vi "Generate Target Compatibility Report.vi"(8 "Error In":errorcluster, 11 "Install LV Data":T2={"SSH Session"=refnum, "Status Log"="", "Detailed Log"="", "Credentials"={"Hostname or IP"="192.168.7.2", "Username"="root", "Password"=""}, "Target Info"={"OS Version"="", "CPU"="", "Systemd Version"="", "Internet Access"=FALSE, "Device Type"="", "LV Installed Ver"="", "LV Available Ver"="", "LV Upgrade Available"=FALSE, "Hostname"="", "NIC Info"=[]}, "Reboot Required?"=FALSE}) -> (0 "Error Out":errorcluster, 1 "Can Continue?":bool, 2 "Warnings":T1[](array[typedef]), 3 "Install LV Data":T2={"SSH Session"=refnum, "Status Log"="", "Detailed Log"="", "Credentials"={"Hostname or IP"="192.168.7.2", "Username"="root", "Password"=""}, "Target Info"={"OS Version"="", "CPU"="", "Systemd Version"="", "Internet Access"=FALSE, "Device Type"="", "LV Installed Ver"="", "LV Available Ver"="", "LV Upgrade Available"=FALSE, "Hostname"="", "NIC Info"=[]}, "Reboot Required?"=FALSE})   [LabVIEW 2014, in "LMH-LINX.lvlib"]
uses:
  <vilib>/MakerHub/LINX/LMH-LINX.lvlib
  <vilib>/MakerHub/LINX/Private/Utilties/Target Management/Install LV Data.ctl
  C:/Program Files (x86)/National Instruments/LabVIEW 2014/vi.lib/MakerHub/LINX/Resources/Renci.SshNet.dll
  Resources/Renci.SshNet.dll
  <vilib>/MakerHub/LINX/Private/Utilties/Target Management/Target Info.ctl
  <vilib>/MakerHub/LINX/Private/Utilties/Target Management/NIC Info.ctl
  <vilib>/MakerHub/LINX/Private/Utilties/Target Management/NIC Mode.ctl
  <vilib>/MakerHub/LINX/Private/Utilties/Target Management/Target Compatibility Warnings.ctl
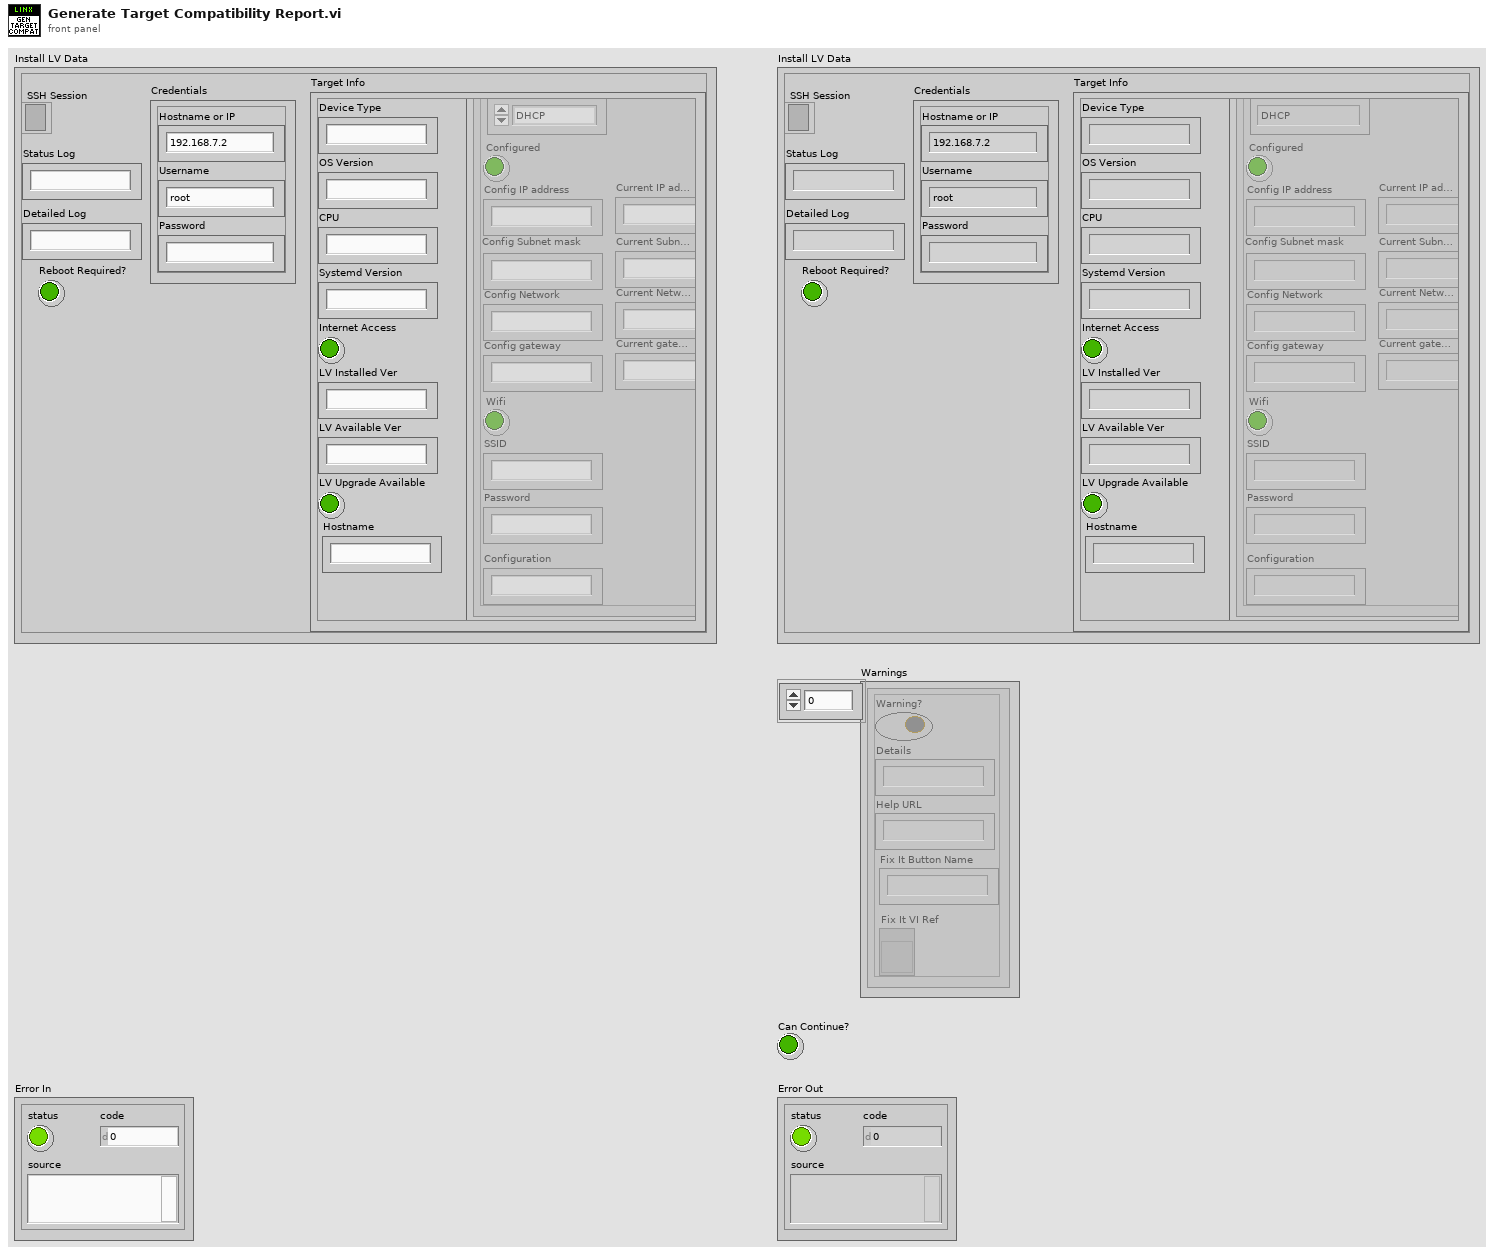
[diagram p1: front panel]
types:
  T1 = typedef "LMH-LINX.lvlib/Target Compatibility Warnings.ctl" = cluster{"Warning?":bool, "Details":string, "Help URL":string, "Fix It Button Name":string, "Fix It VI Ref":refnum<vi>}
  T2 = typedef "LMH-LINX.lvlib/Install LV Data.ctl" = cluster{"SSH Session":refnum<k24>, "Status Log":string, "Detailed Log":string, "Credentials":cluster{"Hostname or IP":string, "Username":string, "Password":string}, "Target Info":T3, "Reboot Required?":bool}
  T3 = typedef "LMH-LINX.lvlib/Target Info.ctl" = cluster{"OS Version":string, "CPU":string, "Systemd Version":string, "Internet Access":bool, "Device Type":string, "LV Installed Ver":string, "LV Available Ver":string, "LV Upgrade Available":bool, "Hostname":string, "NIC Info":T4[]}
  T4 = typedef "LMH-LINX.lvlib/NIC Info.ctl" = cluster{"Name":string, "NIC Mode":T5, "Configured":bool, "Config IP address":string, "Config Subnet mask":string, "Config Network":string, "Config gateway":string, "Wifi":bool, "SSID":string, "Password":string, "Configuration":string, "Current IP address":string, "Current Subnet mask":string, "Current gateway":string, "Current Network":string}
  T5 = typedef "LMH-LINX.lvlib/NIC Mode.ctl" = enum16{"DHCP", "Static", "Loopback"}
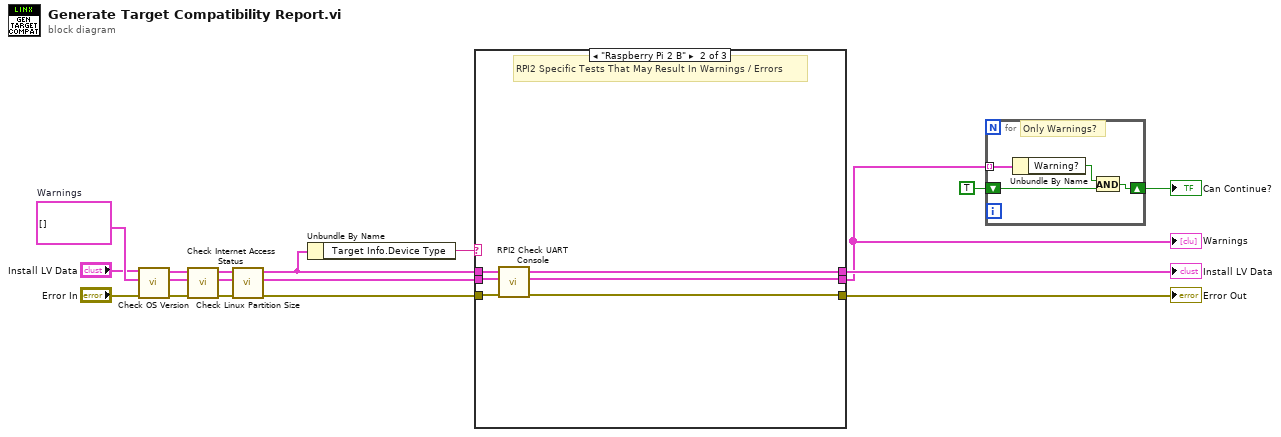
[diagram p0: block diagram]
diagram:
  w17 = T1[] []  # Warnings
  n1 = call <vilib>:"Check OS Version.vi"("Error In"="Error In", "Warnings in"=w17, "Install LV Data"="Install LV Data") -> ("Error Out"=w14:errorcluster, "Warnings"=w12:T1[], "Install LV Data"=w10:T2)  [unwired: 6 in]
  n2 = call <vilib>:"Check Internet Access Status.vi"("Error In"=w14, "Warnings in"=w12, "Install LV Data"=w10) -> ("Error Out"=w4:errorcluster, "Warnings out"=w5:T1[], "Install LV Data"=w6:T2)  [unwired: 6 in]
  n3 = call <vilib>:"Check Linux Partition Size.vi"("Error In"=w4, "Warnings"=w5, "Install LV Data"=w6) -> ("Error Out"=w3:errorcluster, "Warnings"=w1:T1[], "Install LV Data"=w2:T2)  [unwired: 6 in]
  n4 = Unbundle By Name(w2) -> ("Target Info.Device Type"=w9:string)
  n5 = case shown="\"Raspberry Pi 2 B\"" w9 {
    tunnel: w3 -> [w20 w25 w30]
    tunnel: [w20 w24 w30] -> w13
    tunnel: w1 -> [w21 w26 w29]
    tunnel: w2 -> [w19 w27 w28]
    tunnel: [w21 w22 w29] -> w7
    tunnel: [w19 w23 w28] -> w8
    frame Default {
      # "Device Specific Checks"
    }
    frame "Raspberry Pi 2 B" {
      # "RPI2 Specific Tests That May Result In Warnings / Errors"
      n6 = call <vilib>:"RPI2 Check UART Console.vi"("Error In"=w25, "Warnings"=w26, "Install LV Data"=w27) -> ("Error Out"=w24:errorcluster, "Warnings"=w22:T1[], "Install LV Data"=w23:T2)  [unwired: 6 in]
    }
    frame "BeagleBone Black" {
      # "BB Black Specific Tests That May Result In Warnings / Errors"
    }
  }
  "Install LV Data" <- w8
  "Warnings" <- w7
  "Error Out" <- w13
  n7 = for {
    shift-right: [w32] -> w15
    shift-left: TRUE -> [w34]
    tunnel: w7 -> [w31] mode=indexing
    # "Only Warnings?"
    n8 = Unbundle By Name(w31) -> ("Warning?"=w33:bool)
    n9 = And(x=w33, y=w34) -> (x .and. y?=w32:bool)
  }
  "Can Continue?" <- w15
